vi "Countdown_subVI_BM.vi"(10 "Current Iteration":i32, 11 "Runtime (min)":dbl) -> (0 "Global Stop":bool, 3 "Countdown Timer (min)":dbl=-0.00078125 format="%.2g")   [LabVIEW 2021]
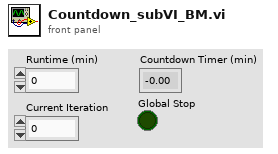
[diagram p1: front panel]
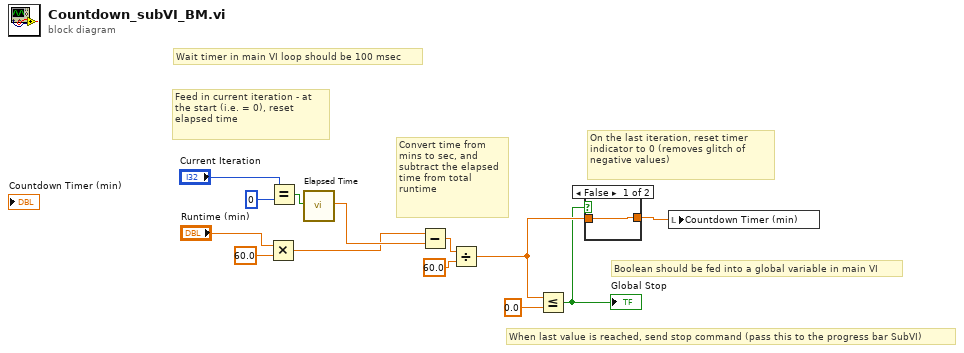
[diagram p0: block diagram]
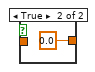
[diagram p2: hidden frame]
diagram:
  # "Wait timer in main VI loop should be 100 msec"
  # "When last value is reached, send stop command (pass this to the progress bar SubVI)"
  # "Convert time from mins to sec, and subtract the elapsed time from total runtime"
  # "Boolean should be fed into a global variable in main VI"
  # "Feed in current iteration - at the start (i.e. = 0), reset elapsed time"
  # "On the last iteration, reset timer indicator to 0 (removes glitch of negative values)"
  n1 = Multiply(x="Runtime (min)", y=60.0) -> (x*y=w2:dbl)
  n2 = Equal?(x="Current Iteration", y=0) -> (x = y?=w9:bool)
  n3 = call "Elapsed Time"("Reset"=w9) -> ("Elapsed Time (s)"=w10:dbl)  [unwired: 11 in, 7 out]
  n4 = Subtract(x=w2, y=w10) -> (x-y=w8:dbl)
  n5 = Divide(x=w8, y=60.0) -> (x/y=w12:dbl)
  n6 = Less Or Equal?(x=w12, y=0.0) -> (x <= y?=w11:bool)
  "Global Stop" <- w11
  n7 = case shown="False" w11 {
    tunnel: [w14 0.0 ("y")] -> w13
    tunnel: w12 -> [w14 _]
    frame False {
    }
    frame True {
    }
  }
  n8 = local write "Countdown Timer (min)"(w13) -> ()
